vi "Read IL Action.vi"(11 "Interlock in":refnum<class "Interlock.lvclass">) -> (2 "IL Action":refnum<class "IL Action.lvclass">[](array[class]), 3 "Interlock out":refnum<class "Interlock.lvclass">)   [LabVIEW 2015, in "Interlocks.lvlib" / "Interlock.lvclass"]
uses:
  Interlock.lvclass
  IL Action/IL Action.lvclass
  Interlock.lvclass/Interlock.ctl
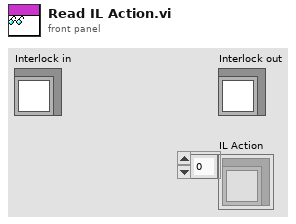
[diagram p1: front panel]
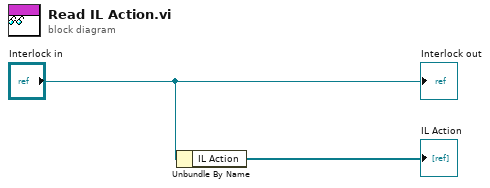
[diagram p0: block diagram]
diagram:
  n1 = Unbundle By Name("Interlock in") -> ("IL Action"=→"IL Action":refnum<class "IL Action.lvclass">[])
  "Interlock out" <- "Interlock in"
